vi "relay board with separate toggles.vi"() -> ()   [LabVIEW 2013]
panel:
  in  "Boolean 1":bool
  in  "Boolean 8":bool
  in  "Boolean 7":bool
  in  "Boolean 6":bool
  in  "Boolean 5":bool
  in  "Boolean 4":bool
  in  "Boolean 3":bool
  in  "Boolean 2":bool
  in  "stop":bool
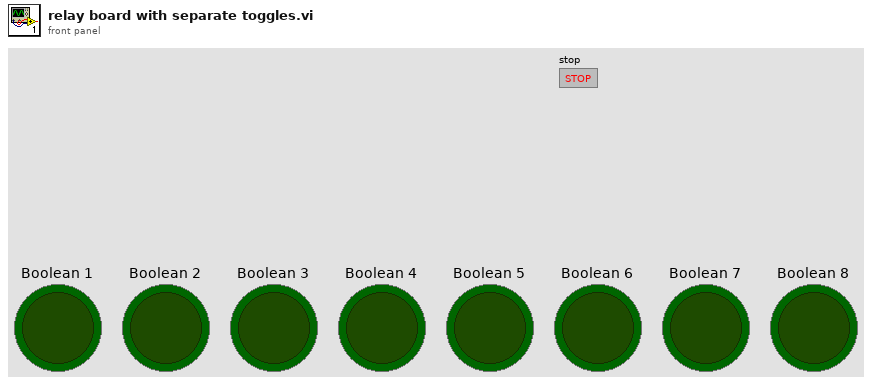
[diagram p1: front panel]
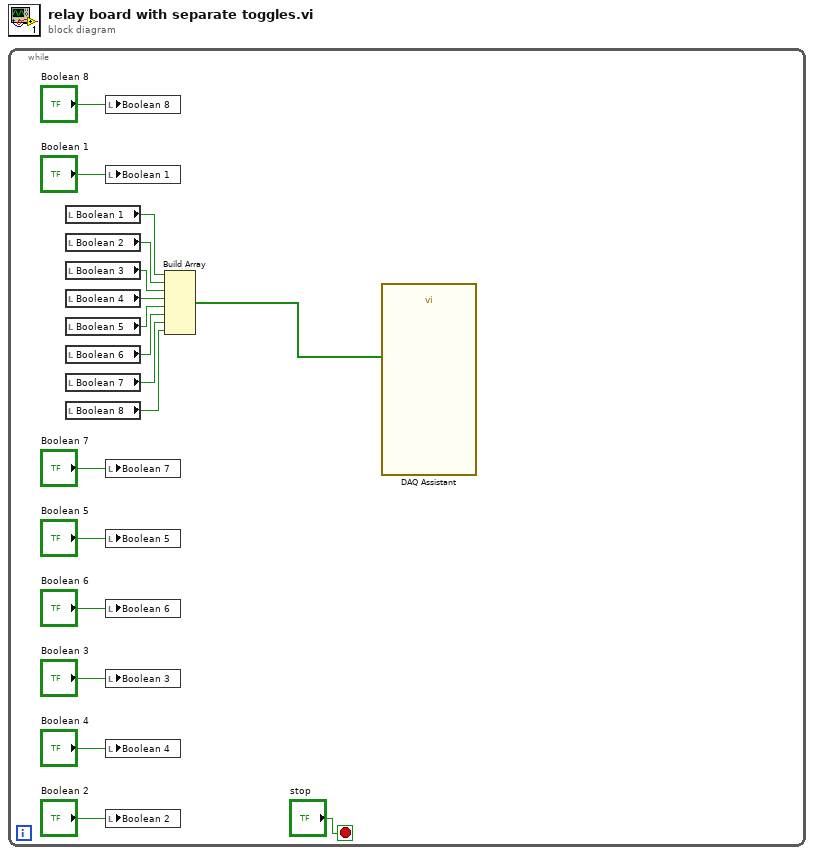
[diagram p0: block diagram]
diagram:
  n1 = while {
    stop <- "stop" stop-if-true
    n2 = local read "Boolean 1"() -> (w17:bool)
    n3 = local read "Boolean 2"() -> (w8:bool)
    n4 = local read "Boolean 3"() -> (w7:bool)
    n5 = local read "Boolean 4"() -> (w6:bool)
    n6 = local read "Boolean 5"() -> (w5:bool)
    n7 = local read "Boolean 6"() -> (w4:bool)
    n8 = local read "Boolean 7"() -> (w3:bool)
    n9 = local read "Boolean 8"() -> (w2:bool)
    n10 = local write "Boolean 8"("Boolean 8") -> ()
    n11 = local write "Boolean 1"("Boolean 1") -> ()
    n12 = local write "Boolean 7"("Boolean 7") -> ()
    n13 = local write "Boolean 5"("Boolean 5") -> ()
    n14 = local write "Boolean 6"("Boolean 6") -> ()
    n15 = local write "Boolean 3"("Boolean 3") -> ()
    n16 = local write "Boolean 4"("Boolean 4") -> ()
    n17 = local write "Boolean 2"("Boolean 2") -> ()
    n18 = Build Array(w17, w8, w7, w6, w5, w4, w3, w2) -> (w1:bool[])
    n19 = call "DAQ Assistant"("data"=w1) -> ()  [unwired: 17 in, 2 out]
  }
